vi "ValidateInput.vi"(8 "error in (no error)":errorcluster, 10 "Input":string, 11 "Code39 in":refnum<class "Code39.lvclass">) -> (0 "error out":errorcluster, 2 "OK":bool=TRUE, 3 "Code39 out":refnum<class "Code39.lvclass">)   [LabVIEW 2013, in "BarCodes.lvlib" / "Code39.lvclass"]
doc: "Returns whether the specified input can be expressed in this barcode format. For Code 39, this will return true if all the characters are in [a-zA-Z0-9. $/+%*-]. Code 39 can represent only capital letters, but this accepts lowercase letters because they get capitialized."
uses:
  Code39.lvclass
  Code39.lvclass/Code39.ctl
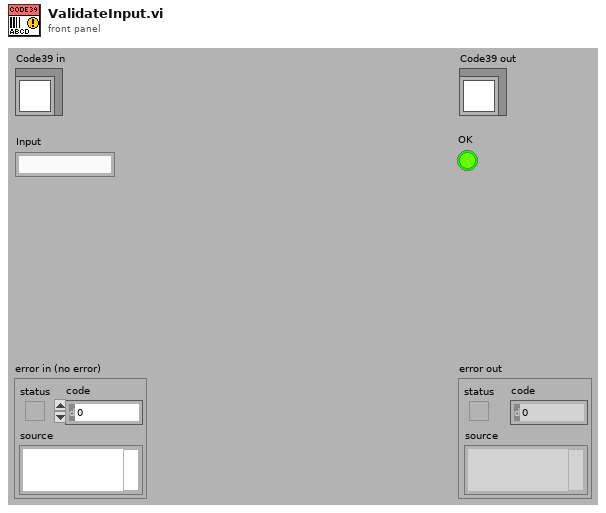
[diagram p1: front panel]
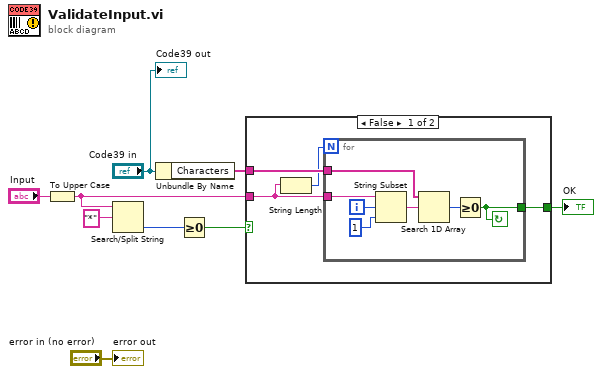
[diagram p0: block diagram]
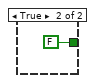
[diagram p2: hidden frame]
diagram:
  n1 = To Upper Case(1:"Input") -> (0:w1:string)
  n2 = Search/Split String(string=w1, search string/char (-)="*") -> (offset of match=w6:i32)  [unwired: 1 in, 2 out]
  n3 = Unbundle By Name("Code39 in") -> ("Characters"=w2:string[])
  n4 = Greater Or Equal To 0?(x=w6) -> (x >= 0?=w5:bool)
  n5 = case shown="False" w5 {
    tunnel: [w10 FALSE] -> w4
    tunnel: w1 -> [w11 _]
    tunnel: w2 -> [w13 _]
    frame False {
      n6 = String Length(string=w11) -> (length=w12:i32)
      n7 = for {
        N: w12 -> [_]
        tunnel: w11 -> [w20]
        tunnel: w13 -> [w17]
        tunnel: [w14] -> w10
        i -> [w19]
        stop <- w14 continue-if-true
        n8 = String Subset(string=w20, offset (0)=w19, length (rest)=1 ("length (rest)")) -> (substring=w16:string)
        n9 = Search 1D Array(1D array=w17, element=w16) -> (index of element=w15:i32)  [unwired: 1 in]
        n10 = Greater Or Equal To 0?(x=w15) -> (x >= 0?=w14:bool)
      }
    }
    frame True {
    }
  }
  "OK" <- w4
  "error out" <- "error in (no error)"
  "Code39 out" <- "Code39 in"
